vi "Register gRPC Methods.vi"(8 "error in (no error)":errorcluster, 11 "Template Server in":refnum<class "GreeterService.lvclass">) -> (0 "error out":errorcluster, 3 "Template Server out":refnum<class "GreeterService.lvclass">)   [LabVIEW 2019, in "Generated_server.lvlib" / "GreeterService.lvclass"]
uses:
  GreeterService.lvclass
  typeDefs/Server Internal UEs.ctl
  typeDefs/Server Internal Message.ctl
  typeDefs/Server gRPC UEs.ctl
  <vilib>/gRPC/LabVIEW gRPC Library/Server API/typeDefs/gRPCId Cluster.ctl
  <vilib>/gRPC/LabVIEW gRPC Library/Shared/grpcId.ctl
  GreeterService.lvclass/GreeterService.ctl
  <vilib>/gRPC/LabVIEW gRPC Library/grpc-lvsupport-release.lvlib
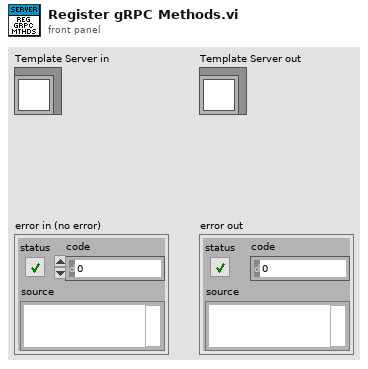
[diagram p1: front panel]
types:
  T1 = typedef "Generated_server.lvlib/GreeterService.lvclass/Server gRPC UEs.ctl" = cluster{"GreeterService SayHello gRPC UE":refnum<user-event>}
  T2 = typedef "Generated_server.lvlib/GreeterService.lvclass/Server Internal UEs.ctl" = cluster{"GreeterService SayHello Internal UE":refnum<user-event>}
  T3 = typedef "grpc-lvsupport-release.lvlib/grpcId.ctl" = u64
  T4 = typedef "Generated_server.lvlib/GreeterService.lvclass/Server Internal Message UE.ctl" = refnum<user-event>
  T5 = typedef "grpc-lvsupport-release.lvlib/gRPCId Cluster UE.ctl" = refnum<user-event>
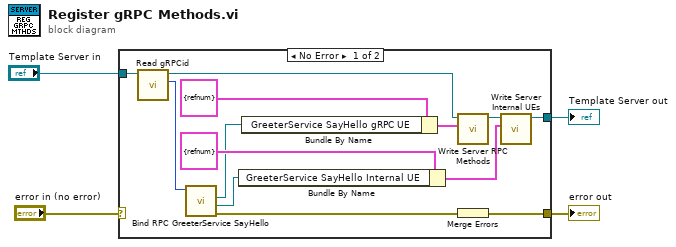
[diagram p0: block diagram]
diagram:
  n1 = case shown="No Error" "error in (no error)" {
    selector: "error in (no error)" -> [_ w18]
    tunnel: "Template Server in" -> [w9 w19]
    tunnel: [w17 w18] -> w3
    tunnel: [w16 w19] -> w2
    frame No Error {
      n2 = call-dynamic "Read gRPCid.vi"("iService in"=w9) -> ("gRPCid"=w8:T3, "iService out"=w10:refnum<class "GreeterService.lvclass">)  [unwired: 8 in, 1 out]
      n3 = call "Bind RPC GreeterService SayHello.vi"("gRPCid server in"=w8) -> ("error out"=w7:errorcluster, "GreeterService SayHello Internal UE"=w5:T4, "GreeterService SayHello gRPC UE"=w6:T5)  [unwired: 7 in, 1 out]
      n4 = Bundle By Name ("Bundle Internal UEs")(cluster=T2 {"GreeterService SayHello Internal UE"=refnum} ("Server Internal UEs"), "GreeterService SayHello Internal UE"=w5) -> (w15:T2)
      n5 = Bundle By Name ("Bundle gRPC UEs")(cluster=T1 {"GreeterService SayHello gRPC UE"=refnum} ("gRPC Server Method Events"), "GreeterService SayHello gRPC UE"=w6) -> (w12:T1)
      n6 = call "Write Server RPC Methods.vi"("Server RPC Methods"=w12, "SignalGeneratorService in"=w10) -> ("SignalGeneratorService out"=w13:refnum<class "GreeterService.lvclass">)  [unwired: 8 in, 1 out]
      n7 = Merge Errors(w7) -> (w17:errorcluster)
      n8 = call "Write Server Internal UEs.vi"("Server Internal UEs"=w15, "SignalGeneratorService in"=w13) -> ("SignalGeneratorService out"=w16:refnum<class "GreeterService.lvclass">)  [unwired: 8 in, 1 out]
    }
    frame Error {
    }
  }
  "error out" <- w3
  "Template Server out" <- w2
